vi "6220_N采样.vi"(2 "率":dbl=10.0, 3 "采样数":i32=10, 4 "timeout (s)":dbl=10.0 caption="超时(s)" format="%0.2f", 5 "error in":errorcluster caption="错误输入", 10 "设备名":tag="6220") -> (16 "6220":cluster{"时间":timestamp, "数据":sgl[][]}, 19 "error out":errorcluster caption="错误输出")   [LabVIEW 2014]
doc: "通过NI-DAQmx创建、编辑和运行任务。关于NI-DAQmx支持设备的完整列表，见NI-DAQ自述文件。\n\n在程序框图上放置DAQ助手Express VI，可通过DAQ助手新建任务。创建任务后，双击DAQ助手Express VI可编辑该任务。如需连续进行测量或信号生成，可将DAQ助手Express VI置于While循环内。"
uses:
  <vilib>/DAQmx/read.llb/DAQmx Read.vi
  <vilib>/DAQmx/read.llb/DAQmx Read (Analog 2D DBL NChan NSamp).vi
  <vilib>/DAQmx/miscellaneous.llb/DAQmx Fill In Error Info.vi
  <vilib>/DAQmx/configure/timing.llb/DAQmx Timing (Sample Clock).vi
  <vilib>/DAQmx/create/channels.llb/DAQmx Create Channel (AI-Voltage-Basic).vi
  <vilib>/DAQmx/create/channels.llb/DAQmx Create Channel (TEDS-AI-Voltage-Basic).vi
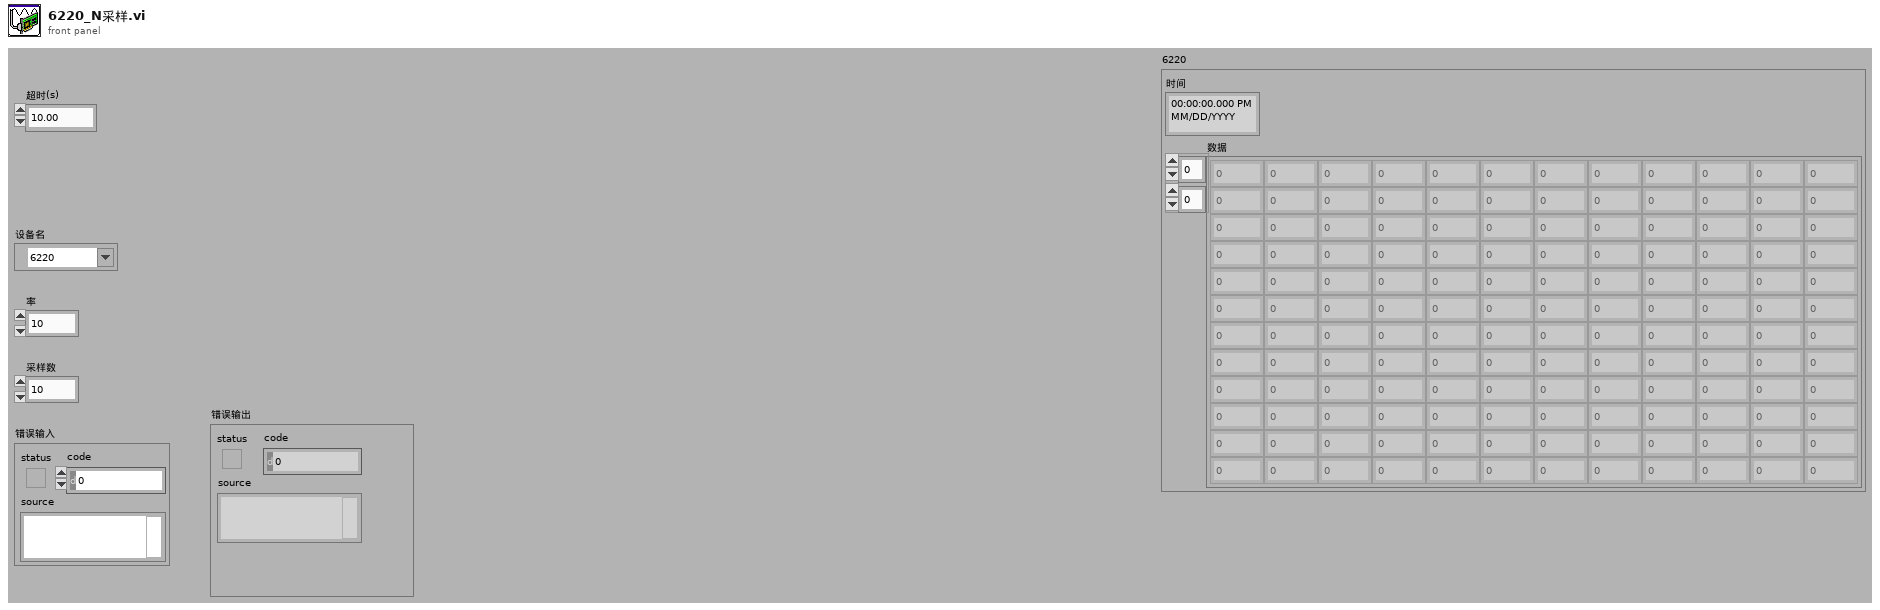
[diagram p1: front panel]
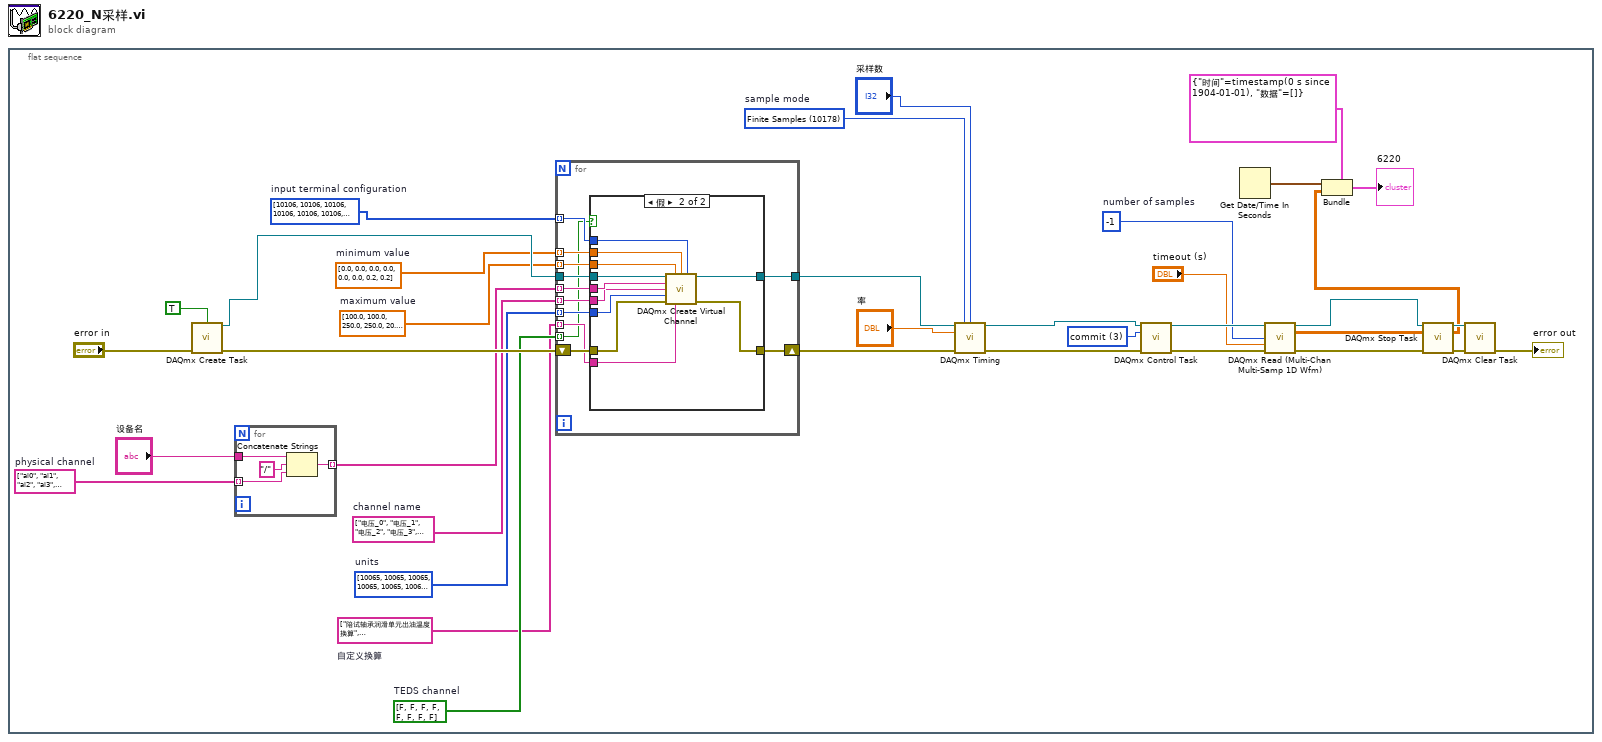
[diagram p0: block diagram]
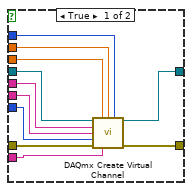
[diagram p2: hidden frame]
diagram:
  n1 = flat-sequence {
    frame #0 {
      w5 = i32[] [10106, 10106, 10106, 10106, 10106, 10106, 10106, 10106] items=["default"=-1, "RSE"=10083, "NRSE"=10078, "Differential"=10106, "Pseudodifferential"=12529]  # input terminal configuration
      w6 = dbl[] [0.0, 0.0, 0.0, 0.0, 0.0, 0.0, 0.2, 0.2]  # minimum value
      w7 = dbl[] [100.0, 100.0, 250.0, 250.0, 20.0, 20.0, 7.0, 7.0]  # maximum value
      w8 = string[] ["陪试轴承润滑单元出油温度换算", "陪试轴承润滑单元出油温度换算", "轴承外圈温度换算", "轴承外圈温度换算", "摩擦力换算", "摩擦力换算", "油缸力换算", "油缸力换算"]  # 自定义换算
      w9 = i32[] [10065, 10065, 10065, 10065, 10065, 10065, 10065, 10065] items=["Volts"=10348, "From TEDS"=12516, "From Custom Scale"=10065]  # units
      w10 = string[] ["电压_0", "电压_1", "电压_2", "电压_3", "电压_4", "电压_5", "电压_6", "电压_7"]  # channel name
      w13 = 3 items=["verify"=2, "reserve"=4, "commit"=3, "unreserve"=5, "abort"=6] ("action")
      w18 = -1  # number of samples
      w23 = 10178 items=["Finite Samples"=10178, "Continuous Samples"=10123, "Hardware Timed Single Point"=12522]  # sample mode
      w28 = bool[] [FALSE, FALSE, FALSE, FALSE, FALSE, FALSE, FALSE, FALSE]  # TEDS channel
      w32 = string[] ["ai0", "ai1", "ai2", "ai3", "ai4", "ai5", "ai6", "ai7"]  # physical channel
      n2 = call <vilib>:"DAQmx Create Task.vi"("auto cleanup"=TRUE, "error in"="error in") -> ("task out"=w31:refnum<k21>, "error out"=w30:errorcluster)  [unwired: 12 in]
      n3 = for "For循环" {
        tunnel: [w39] -> w29 mode=indexing
        tunnel: "设备名" -> [w38]
        tunnel: w32 -> [w36] mode=indexing
        n4 = Concatenate Strings(w38, "/" ("string"), w36) -> (w39:string)
      }
      n5 = for "For循环" {
        tunnel: w31 -> [w51]
        tunnel: [w49] -> w27
        tunnel: w5 -> [w47] mode=indexing
        tunnel: w6 -> [w46] mode=indexing
        tunnel: w7 -> [w45] mode=indexing
        tunnel: w29 -> [w44] mode=indexing
        tunnel: w10 -> [w43] mode=indexing
        tunnel: w9 -> [w42] mode=indexing
        tunnel: w8 -> [w41] mode=indexing
        shift-right: [w48] -> w26
        shift-left: w30 -> [w50]
        tunnel: w28 -> [w40] mode=indexing
        n6 = case "条件结构" shown="假" w40 {
          tunnel: w51 -> [w62 w73]
          tunnel: w50 -> [w61 w72]
          tunnel: [w60 w71] -> w49
          tunnel: [w59 w63] -> w48
          tunnel: w47 -> [w58 w70]
          tunnel: w46 -> [w57 w69]
          tunnel: w45 -> [w56 w68]
          tunnel: w44 -> [w55 w67]
          tunnel: w43 -> [w54 w66]
          tunnel: w42 -> [w53 w65]
          tunnel: w41 -> [w52 w64]
          frame True {
            n7 = call-poly <vilib>:"DAQmx Create Virtual Channel.vi"("task in"=w62, "maximum value"=w56, "minimum value"=w57, "input terminal configuration"=w58, "physical channels"=w55, "name to assign"=w54, "units"=w53, "error in"=w61, "custom scale name"=w52) -> ("task out"=w60:refnum<k21>, "error out"=w59:errorcluster)  [unwired: 5 in]
          }
          frame False {
            n8 = call-poly <vilib>:"DAQmx Create Virtual Channel.vi"("task in"=w73, "maximum value"=w68, "minimum value"=w69, "input terminal configuration"=w70, "physical channels"=w67, "name to assign"=w66, "units"=w65, "error in"=w72, "custom scale name"=w64) -> ("task out"=w71:refnum<k21>, "error out"=w63:errorcluster)  [unwired: 5 in]
          }
        }
      }
      n9 = call-poly <vilib>:"DAQmx Timing.vi"("task/channels in"=w27, "sample mode"=w23, "samples per channel"="采样数", "rate"="率", "error in"=w26) -> ("task out"=w22:refnum<k21>, "error out"=w21:errorcluster)  [unwired: 9 in]
      n10 = call <vilib>:"DAQmx Control Task.vi"("task/channels in"=w22, "action"=w13, "error in"=w21) -> ("task out"=w20:refnum<k21>, "error out"=w19:errorcluster)  [unwired: 11 in]
      n11 = Get Date/Time In Seconds() -> (seconds since 1Jan1904=w4:timestamp)
      n12 = call-poly "DAQmx Read (Multi-Chan Multi-Samp 1D Wfm).vi"("task/channels in"=w20, "number of samples per channel"=w18, "timeout"="timeout (s)", "error in"=w19) -> ("task out"=w16:refnum<k21>, "data"=w1:dbl[][], "error out"=w15:errorcluster)  [unwired: 9 in]
      n13 = Bundle(cluster=cluster{"时间":timestamp, "数据":sgl[][]} {"时间"=timestamp(0 s since 1904-01-01), "数据"=[]}, "时间"=w4, "数据"=w1) -> (→"6220":cluster{"时间":timestamp, "数据":sgl[][]})
      n14 = call <vilib>:"DAQmx Stop Task.vi"("task/channels in"=w16, "error in"=w15) -> ("task out"=w11:refnum<k21>, "error out"=w12:errorcluster)  [unwired: 12 in]
      n15 = call <vilib>:"DAQmx Clear Task.vi"("task in"=w11, "error in"=w12) -> ("error out"=→"error out":errorcluster)  [unwired: 13 in]
    }
  }
